vi "create Gamry data file v3.vi"(4 "error in":errorcluster, 5 "Extension":string=".txt", 6 "temp":dbl, 7 "dir path":path) -> (0 "error out":errorcluster, 1 "Tempout":i32, 2 "ExpDateTempStr":string, 3 "refnum out":refnum<file>)   [LabVIEW 2018]
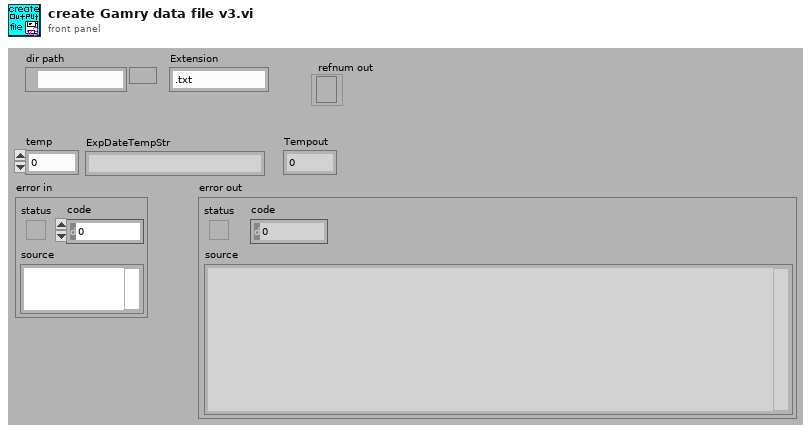
[diagram p1: front panel]
types:
  T1 = enum16{"open", "replace", "create", "open or create", "replace or create", "replace or create with confirmation"}
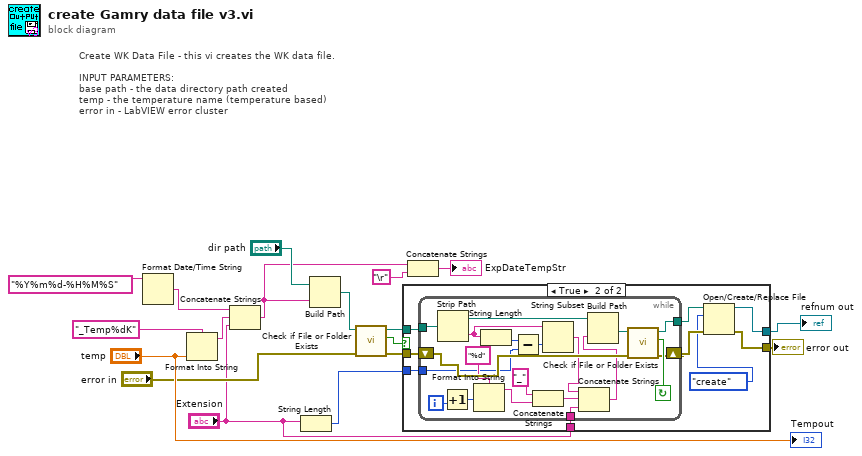
[diagram p0: block diagram]
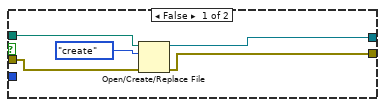
[diagram p2: hidden frame]
diagram:
  # "Create WK Data File - this vi creates the WK data file.\n\nINPUT PARAMETERS:\nbase path - the data directory path created\ntemp - the temperature name (temperature based)\nerror in - LabVIEW error cluster"
  n1 = Format Date/Time String(time format string (%c)="%Y%m%d-%H%M%S") -> (date/time string=w13:string)  [unwired: 2 in]
  n2 = Format Into String(format string="_Temp%dK", "temp") -> (resulting string=w8:string)  [unwired: 2 in, 1 out]
  n3 = Concatenate Strings(w13, w8, "Extension") -> (w9:string)
  n4 = String Length(string="Extension") -> (length=w2:i32)
  n5 = Build Path(base path="dir path", name or relative path=w9) -> (appended path=w7:path)
  n6 = call <vilib>:"Check if File or Folder Exists.vi"("error in (no error)"="error in", "path"=w7) -> ("error out"=w4:errorcluster, "file or folder exists?"=w3:bool, "dup path"=w6:path)  [unwired: 7 in]
  n7 = case shown="True" w3 {
    tunnel: [w21 w29] -> w18
    tunnel: [w20 w28] -> w10
    tunnel: w6 -> [w19 w32]
    tunnel: w4 -> [w22 w31]
    tunnel: "Extension" -> [_ w25]
    tunnel: w2 -> [_ w24]
    frame False {
      n8 = Open/Create/Replace File(file path (use dialog)=w19, error in=w22, operation (0:open)=T1."create") -> (refnum out=w20:refnum<file>, error out=w21:errorcluster)  [unwired: 3 in, 1 out]
    }
    frame True {
      n9 = while {
        tunnel: w32 -> [w46]
        shift-right: [w39] -> w27
        shift-left: w31 -> [w52]
        tunnel: [w40] -> w30
        tunnel: w25 -> [w38]
        tunnel: w24 -> [w34]
        i -> [w42]
        stop <- w50 continue-if-true
        n10 = Strip Path(path=w46) -> (stripped path=w45:path, name=w36:string)
        n11 = Increment(x=w42) -> (x+1=w41:i32)
        n12 = Format Into String(format string="%d", w41) -> (resulting string=w48:string)  [unwired: 2 in, 1 out]
        n13 = String Length(string=w36) -> (length=w35:i32)
        n14 = Subtract(x=w35, y=w34) -> (x-y=w33:i32)
        n15 = Concatenate Strings("_", w48) -> (w44:string)
        n16 = String Subset(string=w36, length (rest)=w33) -> (substring=w37:string)  [unwired: 1 in]
        n17 = Concatenate Strings(w37, w44, w38) -> (w43:string)
        n18 = Build Path(base path=w45, name or relative path=w43) -> (appended path=w51:path)
        n19 = call <vilib>:"Check if File or Folder Exists.vi"("error in (no error)"=w52, "path"=w51) -> ("error out"=w39:errorcluster, "file or folder exists?"=w50:bool, "dup path"=w40:path)  [unwired: 7 in]
      }
      n20 = Open/Create/Replace File(file path (use dialog)=w30, error in=w27, operation (0:open)=T1."create") -> (refnum out=w28:refnum<file>, error out=w29:errorcluster)  [unwired: 3 in, 1 out]
    }
  }
  "error out" <- w18
  "refnum out" <- w10
  n21 = Concatenate Strings(w9, "\r") -> (→"ExpDateTempStr":string)
  "Tempout" <- "temp"
